vi "EnumPassing.vi"(10 "Number of Hours Worked":dbl, 11 "Class Standing Input":T1(ring)=enum."Junior") -> (2 "Pay":dbl, 3 "Class Standing Output":T1(ring))   [LabVIEW 2014]
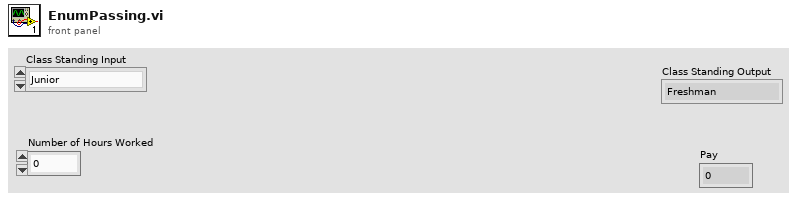
[diagram p1: front panel]
types:
  T1 = enum16{"Freshman", "Sophomore", "Junior", "Senior"}
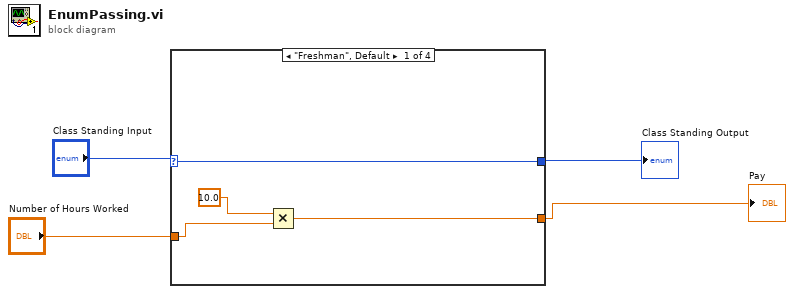
[diagram p0: block diagram]
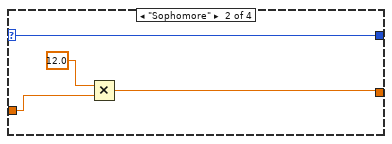
[diagram p2: hidden frame]
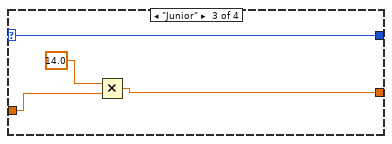
[diagram p3: hidden frame]
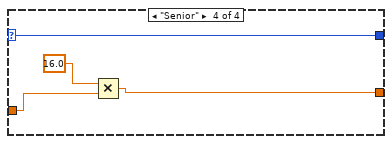
[diagram p4: hidden frame]
diagram:
  n1 = case shown="\"Freshman\", Default" "Class Standing Input" {
    selector: "Class Standing Input" -> [w8 w10 w13 w17]
    tunnel: "Number of Hours Worked" -> [w6 w12 w15 w19]
    tunnel: [w8 w10 w13 w17] -> w2
    tunnel: [w5 w9 w14 w18] -> w1
    frame "Freshman", Default {
      n2 = Multiply(x=10.0 ("Number of Hours Worked"), y=w6) -> (x*y=w5:dbl)
    }
    frame "Sophomore" {
      n3 = Multiply(x=12.0 ("Number of Hours Worked"), y=w12) -> (x*y=w9:dbl)
    }
    frame "Junior" {
      n4 = Multiply(x=14.0 ("Number of Hours Worked"), y=w15) -> (x*y=w14:dbl)
    }
    frame "Senior" {
      n5 = Multiply(x=16.0 ("Number of Hours Worked"), y=w19) -> (x*y=w18:dbl)
    }
  }
  "Pay" <- w1
  "Class Standing Output" <- w2
